vi "Select Symbol.vi"(11 "Hierarchy":string[](array[string])) -> (3 "Symbol ID":string)   [LabVIEW 2020, in "VI Properties Editor.lvlib" / "Tree Map.lvlib" / "Tree Map.lvclass"]
uses:
  Tree Map.lvclass
  Tree Map.lvclass/Tree Map.ctl
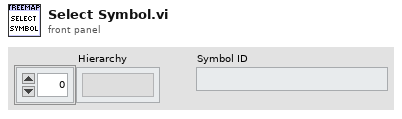
[diagram p1: front panel]
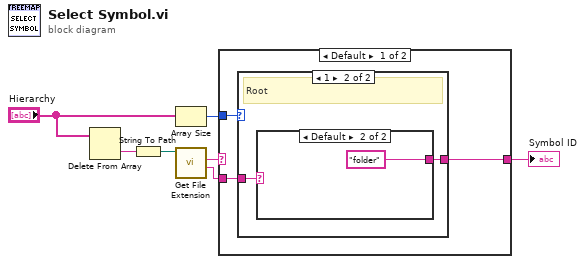
[diagram p0: block diagram]
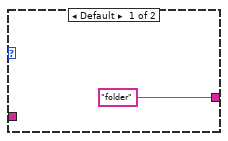
[diagram p2: hidden frame]
diagram:
  n1 = Delete From Array(array="Hierarchy") -> (deleted portion=w2:string)  [unwired: 2 in, 1 out]
  n2 = String To Path(string=w2) -> (path=w3:path)
  n3 = Array Size(array="Hierarchy") -> (size(s)=w6:i32)
  n4 = call <vilib>:"Get File Extension.vi"("file"=w3) -> ("filename without extension"=w5:string, "lowercase file extension"=w4:string)  [unwired: 6 in, 3 out]
  n5 = case shown="Default" w4 {
    selector: w4 -> [_ w16]
    tunnel: [w10 w16] -> w7
    tunnel: w5 -> [w9 _]
    tunnel: w6 -> [w8 _]
    frame Default {
      n6 = case shown="1" w8 {
        tunnel: ["folder" w13] -> w10
        tunnel: w9 -> [_ w12]
        frame Default {
        }
        frame 1 {
          # "Root"
          n7 = case shown="Default" w12 {
            selector: w12 -> [w14 _]
            tunnel: [w14 "folder"] -> w13
            frame "My Computer" {
            }
            frame Default {
            }
          }
        }
      }
    }
    frame "lvclass", "lvlib", "target", "vi", "vim", "vit" {
    }
  }
  "Symbol ID" <- w7
